vi "Load.vi"(8 "error in (no error)":errorcluster, 10 "Model Path":path, 11 "MarkovModel in":refnum<class "MarkovModel.lvclass">) -> (0 "error out":errorcluster, 3 "MarkovModel out":refnum<class "MarkovModel.lvclass">)   [LabVIEW 2020, in "MarkovModel.lvclass"]
uses:
  MarkovModel.lvclass
  MarkovModel.lvclass/MarkovModel.ctl
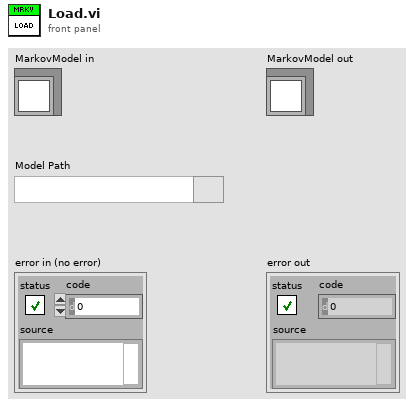
[diagram p1: front panel]
types:
  T1 = map{string[], cluster{"Class Name":string, "Count":i32}[]}
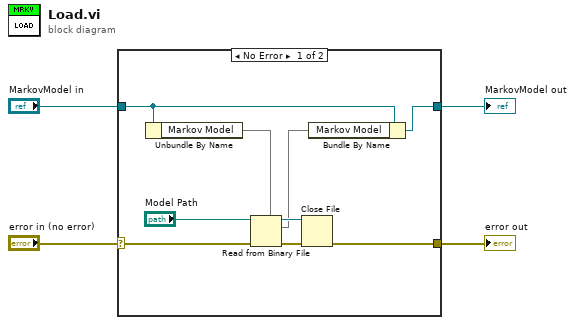
[diagram p0: block diagram]
diagram:
  n1 = case shown="No Error" "error in (no error)" {
    selector: "error in (no error)" -> [w11 w15]
    tunnel: [w10 w15] -> w3
    tunnel: "MarkovModel in" -> [w7 w14]
    tunnel: [w6 w14] -> w1
    frame No Error {
      n2 = Unbundle By Name(w7) -> ("Markov Model"=w8:T1)
      n3 = Read from Binary File(5:w8, 8:w11, 11:"Model Path") -> (0:w13:errorcluster, 2:w5:T1, 3:w12:refnum<file>)  [unwired: 3 in, 1 out]
      n4 = Close File(refnum=w12, error in=w13) -> (error out=w10:errorcluster)  [unwired: 1 out]
      n5 = Bundle By Name(cluster=w7, "Markov Model"=w5) -> (w6:refnum<class "MarkovModel.lvclass">)
    }
    frame Error {
    }
  }
  "error out" <- w3
  "MarkovModel out" <- w1
